vi "Generator Driver Template 3.vi"() -> ()   [LabVIEW 2024]
uses:
  subVIs/Revidyne Generator.lvlib
panel:
  out "Waveform Chart":dbl(graph)
  in  "Speed":dbl(slide) scale=0.0..255.0
  in  "stop":bool
  in  "VISA resource name":refnum<visa-resource-name>
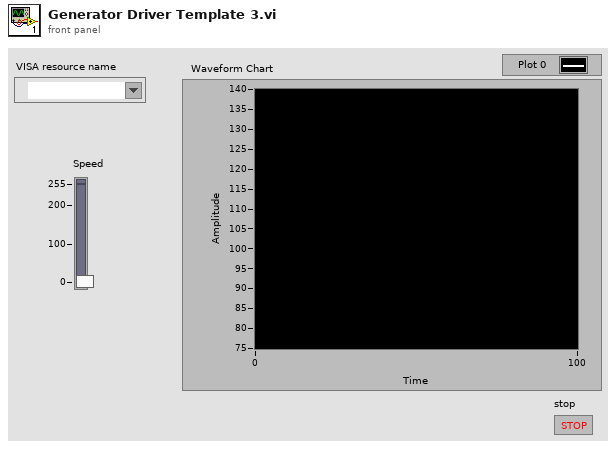
[diagram p1: front panel]
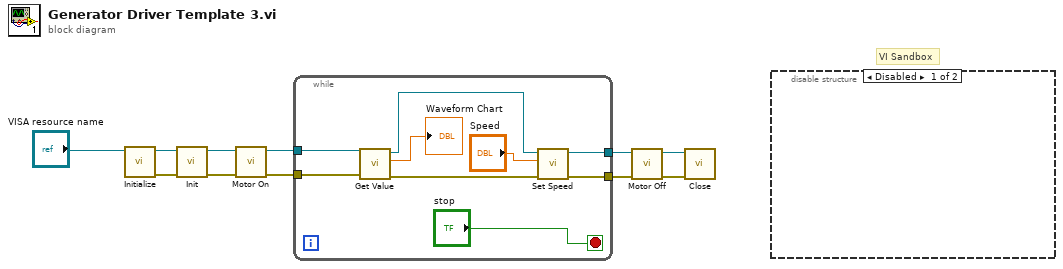
[diagram p0: block diagram]
diagram:
  # "VI Sandbox"
  n1 = call "Initialize.vi"("VISA resource name"="VISA resource name") -> ("error out"=w10:errorcluster, "VISA resource name out"=w11:refnum<visa-resource-name>)  [unwired: 9 in]
  n2 = call "Init.vi"("error in (no error)"=w10, "VISA resource name"=w11) -> ("error out"=w8:errorcluster, "VISA resource name out"=w9:refnum<visa-resource-name>)  [unwired: 8 in]
  n3 = call "Motor On.vi"("error in"=w8, "VISA resource name"=w9) -> ("error out"=w6:errorcluster, "VISA resource name out"=w7:refnum<visa-resource-name>)  [unwired: 8 in]
  n4 = while {
    tunnel: w7 -> [w20]
    tunnel: w6 -> [w19]
    tunnel: [w15] -> w4
    tunnel: [w13] -> w1
    stop <- "stop" stop-if-true
    n5 = call "Get Value.vi"("error in (no error)"=w19, "VISA resource name"=w20) -> ("error out"=w16:errorcluster, "Value"=→"Waveform Chart":dbl, "VISA resource name out"=w14:refnum<visa-resource-name>)  [unwired: 7 in]
    n6 = call "Set Speed.vi"("error in (no error)"=w16, "speed (0)"="Speed", "VISA resource name"=w14) -> ("error out"=w15:errorcluster, "VISA resource name out"=w13:refnum<visa-resource-name>)  [unwired: 7 in]
  }
  n7 = call "Motor Off.vi"("error in (no error)"=w4, "VISA resource name"=w1) -> ("error out"=w3:errorcluster, "VISA resource name out"=w5:refnum<visa-resource-name>)  [unwired: 8 in]
  n8 = call "Close.vi"("error in (no error)"=w3, "VISA resource name"=w5) -> ()  [unwired: 9 in, 1 out]
  n9 = disable-structure shown="Disabled" {
    frame Disabled {
    }
    frame Enabled {
    }
  }
